vi "Get Project Number.vi"(8 "error in (no error)":errorcluster, 11 "Project Number Msg in":refnum<class "Project Number Msg.lvclass">) -> (0 "error out":errorcluster, 2 "Project Number":i32, 3 "Project Number Msg out":refnum<class "Project Number Msg.lvclass">)   [LabVIEW 2013, in "Main Model.lvlib" / "Project Number Msg.lvclass"]
uses:
  Project Number Msg.lvclass
  Project Number Msg.lvclass/Project Number Msg.ctl
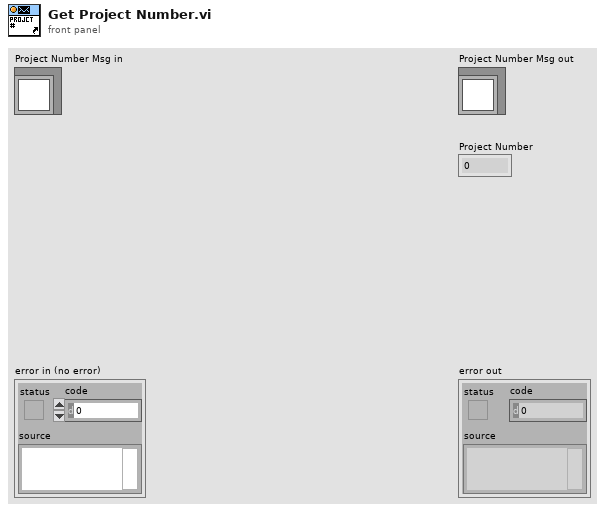
[diagram p1: front panel]
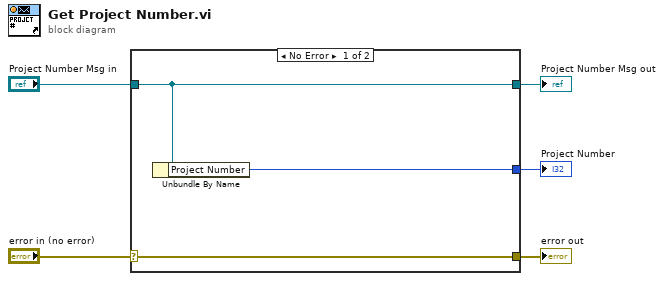
[diagram p0: block diagram]
diagram:
  n1 = case shown="No Error" "error in (no error)" {
    selector: "error in (no error)" -> [w8 w9]
    tunnel: [w8 w9] -> w4
    tunnel: [w7 w10] -> w2
    tunnel: "Project Number Msg in" -> [w7 w10]
    tunnel: [w6 _] -> w1
    frame No Error {
      n2 = Unbundle By Name(w7) -> ("Project Number"=w6:i32)
    }
    frame Error {
    }
  }
  "error out" <- w4
  "Project Number Msg out" <- w2
  "Project Number" <- w1
